vi "Write Scalar Data.vi"(8 "error in (no error)":errorcluster, 9 "Changed?":bool[](array[boolean]), 10 "Values":dbl[](array[numeric]), 11 "Cluster":T1 {"Data Type" format="%.0x"}) -> (0 "error out":errorcluster, 2 "Values":dbl[](array[numeric]), 3 "Cluster":T1 {"Data Type" format="%.0x"})   [LabVIEW 2017, in "FPGA Addon Engine.lvlib"]
uses:
  FPGA Addon Engine.lvlib
  Types/Register Settings.ctl
  Shared/Data Type.ctl
  Shared/Scalar Type.ctl
  <vilib>/rvi/errors/niLvFpgaAdjustHostInterfaceError.vi
  <vilib>/Utility/error.llb/Error Cluster From Error Code.vi
  <vilib>/rvi/interface/nirviReadWriteControl/nirviReadWriteControl.xnode
  <vilib>/rvi/interface/Simulation/niFpgaSimulationCallBeginRW.vi
  NiFpgaLv.dll
  Shared/FPGA Addon Shared.lvlib
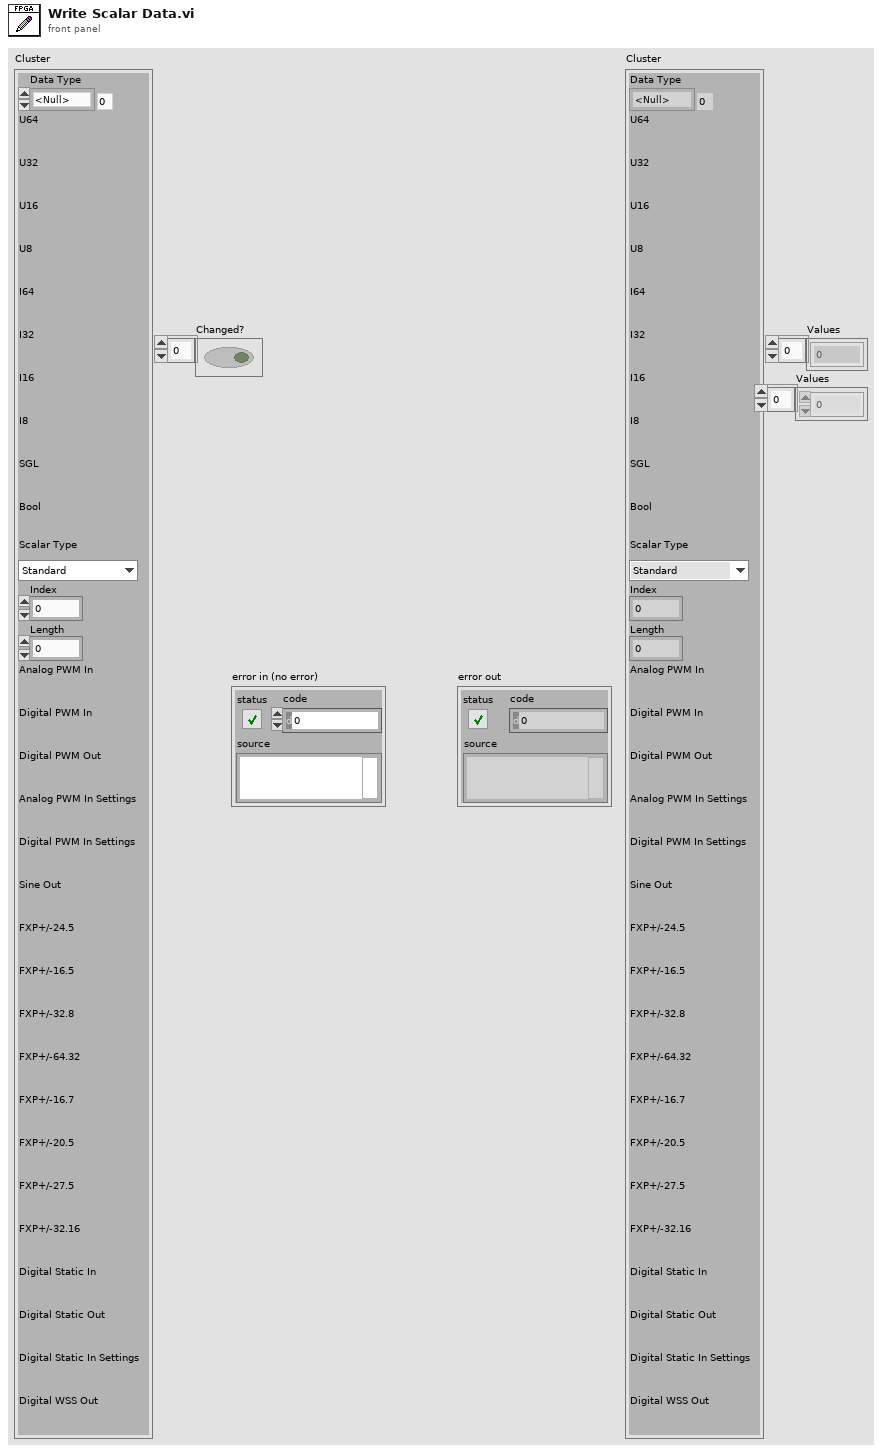
[diagram p1: front panel]
types:
  T1 = typedef "FPGA Addon Engine.lvlib/Register Settings.ctl" = cluster{"Data Type":T2, "U64":refnum<k20>, "U32":refnum<k20>, "U16":refnum<k20>, "U8":refnum<k20>, "I64":refnum<k20>, "I32":refnum<k20>, "I16":refnum<k20>, "I8":refnum<k20>, "SGL":refnum<k20>, "Bool":refnum<k20>, "Scalar Type":T3, "Index":i32, "Length":i32, "Analog PWM In":refnum<k20>, "Digital PWM In":refnum<k20>, "Digital PWM Out":refnum<k20>, "Analog PWM In Settings":refnum<k20>, "Digital PWM In Settings":refnum<k20>, "Sine Out":refnum<k20>, "FXP+/-24.5":refnum<k20>, "FXP+/-16.5":refnum<k20>, "FXP+/-32.8":refnum<k20>, "FXP+/-64.32":refnum<k20>, "FXP+/-16.7":refnum<k20>, "FXP+/-20.5":refnum<k20>, "FXP+/-27.5":refnum<k20>, "FXP+/-32.16":refnum<k20>, "Digital Static In":refnum<k20>, "Digital Static Out":refnum<k20>, "Digital Static In Settings":refnum<k20>, "Digital WSS Out":refnum<k20>}
  T2 = typedef "FPGA Addon Shared.lvlib/Data Type.ctl" = enum8{"<Null>", "I8", "I16", "I32", "I64", "U8", "U16", "U32", "U64", "SGL", "Boolean", "Analog PWM In Settings", "Analog PWM In", "Digital PWM In Settings", "Digital PWM In", "Digital PWM Out", "Sine Out", "FXP+/-24.5", "FXP+/-16.5", "FXP+/-32.8", "FXP+/-64.32", "FXP+/-16.7", "FXP+/-20.5", "FXP+/-27.5", "FXP+/-32.16", "Digital Static In", "Digital Static Out", "Digital Static In Settings", "Digital WSS Out"}
  T3 = typedef "FPGA Addon Shared.lvlib/Scalar Type.ctl" = enum16{"Standard", "Bitpacked"}
  T4 = cluster{"ACTIVE EDGE":bool, "TIMEOUT":u32, "THRESHOLD":fxp<+/-,32,8>}
  T5 = cluster{"ACTIVE EDGE":bool, "ACTIVE TICKS":u32, "INACTIVE TICKS":u32}
  T6 = cluster{"ACTIVE EDGE":bool, "ACTIVE TICKS":u32, "INACTIVE TICKS":u32, "DATA":u8, "SENSOR TYPE":u8}
  T7 = cluster{"AMP":fxp<+/-,32,8>, "OFFSET":fxp<+/-,32,8>, "PERIODS/TICKS":fxp<+,32,0>}
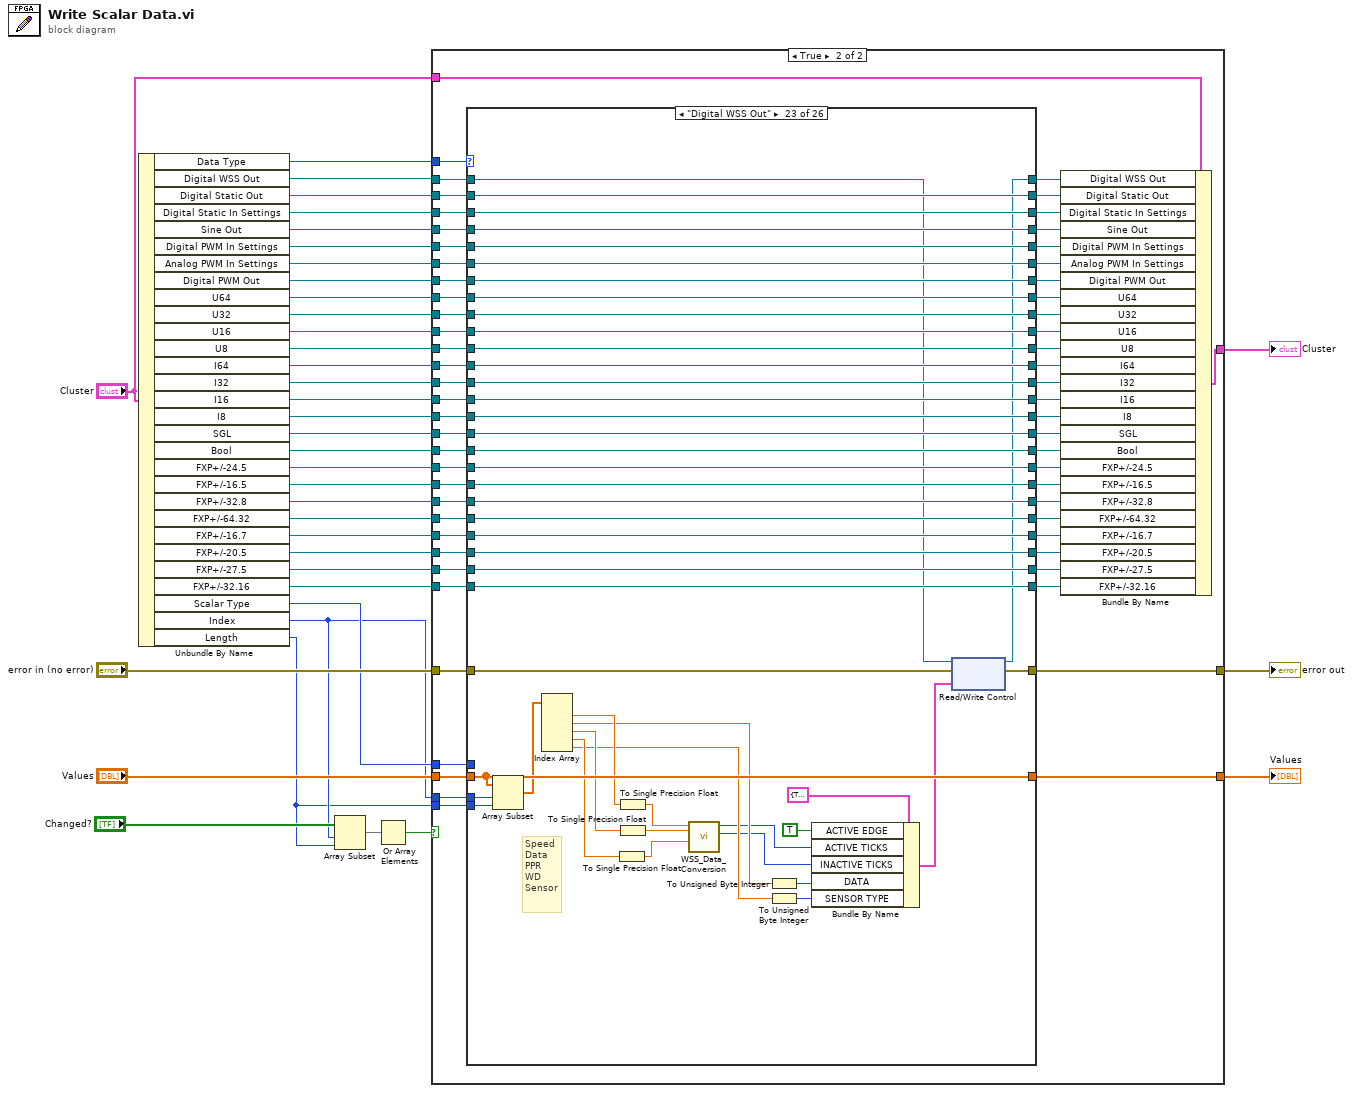
[diagram p0: block diagram]
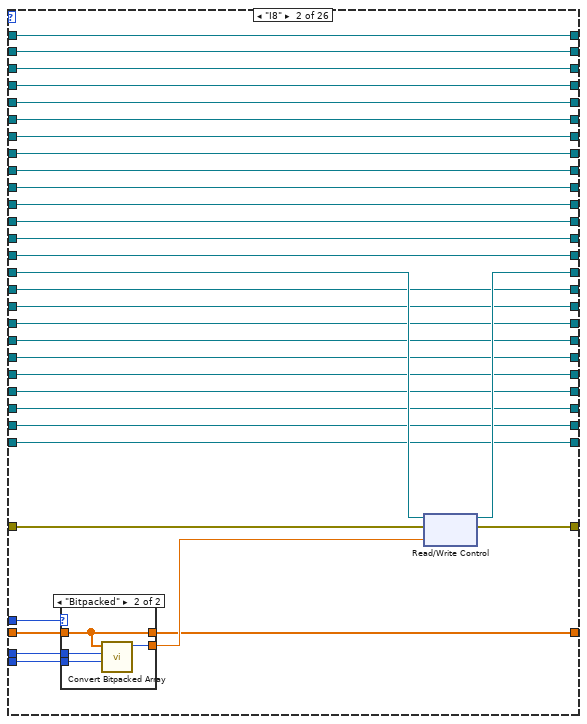
[diagram p4: hidden frame]
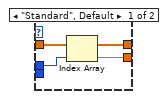
[diagram p5: hidden frame]
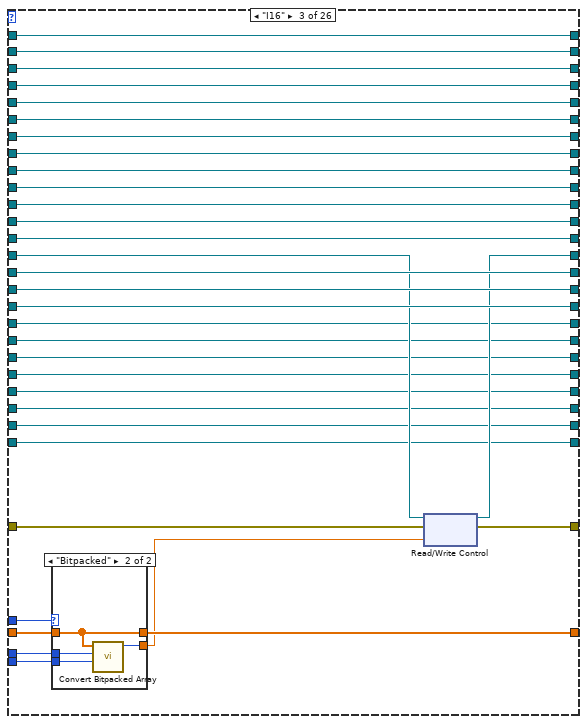
[diagram p6: hidden frame]
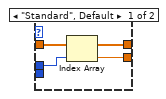
[diagram p7: hidden frame]
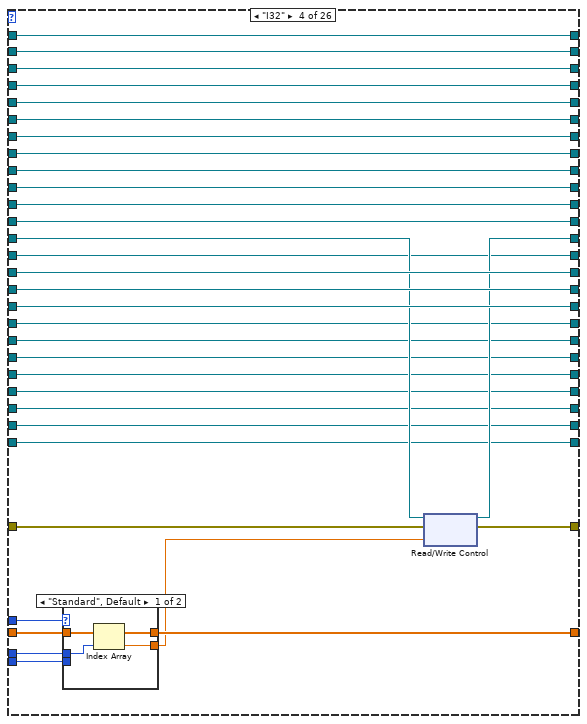
[diagram p8: hidden frame]
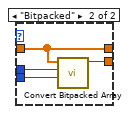
[diagram p9: hidden frame]
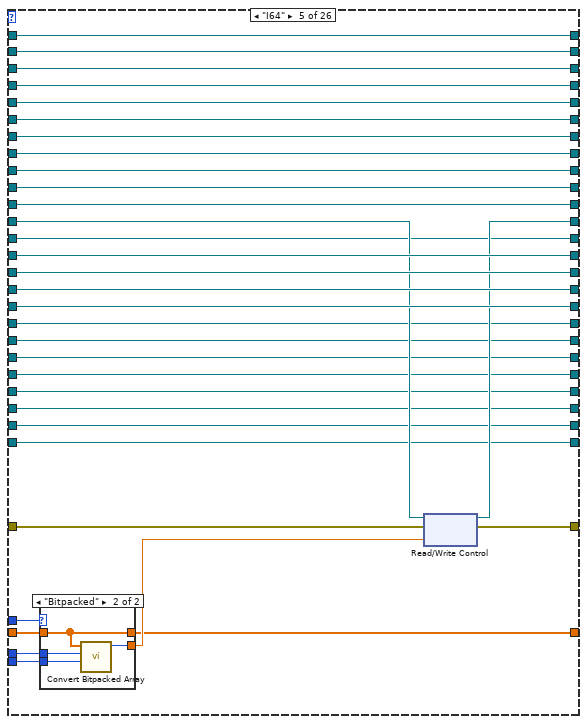
[diagram p10: hidden frame]
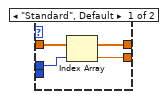
[diagram p11: hidden frame]
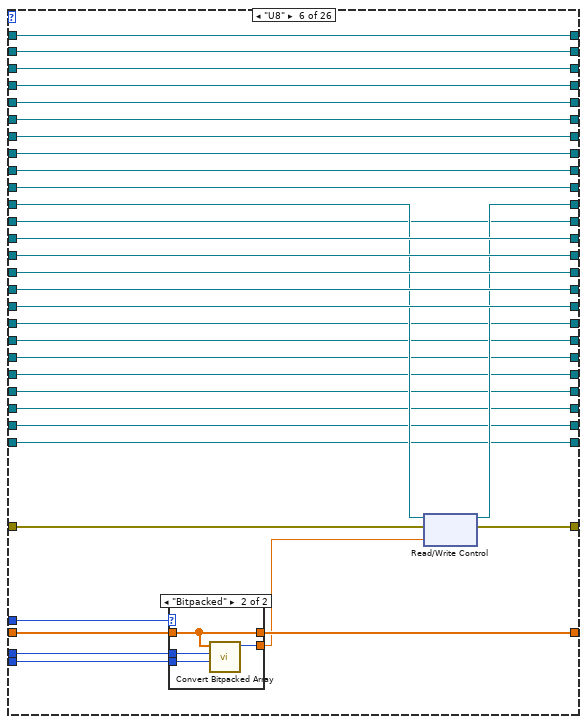
[diagram p12: hidden frame]
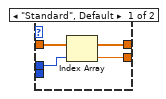
[diagram p13: hidden frame]
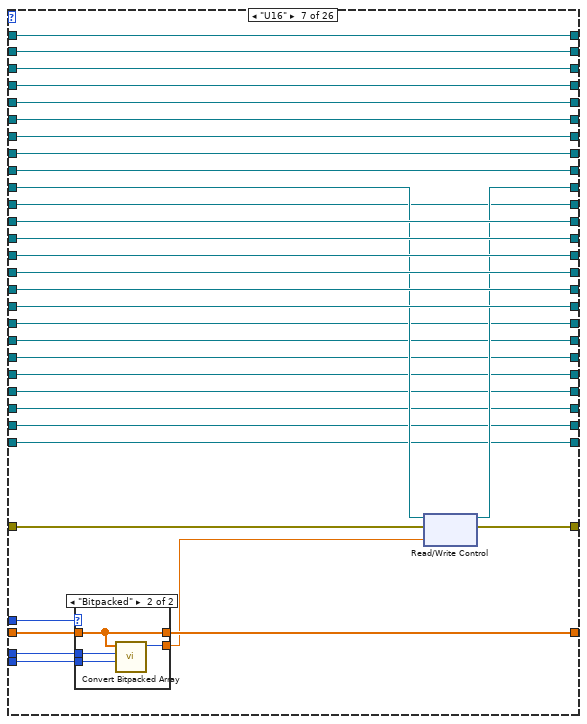
[diagram p14: hidden frame]
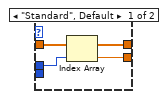
[diagram p15: hidden frame]
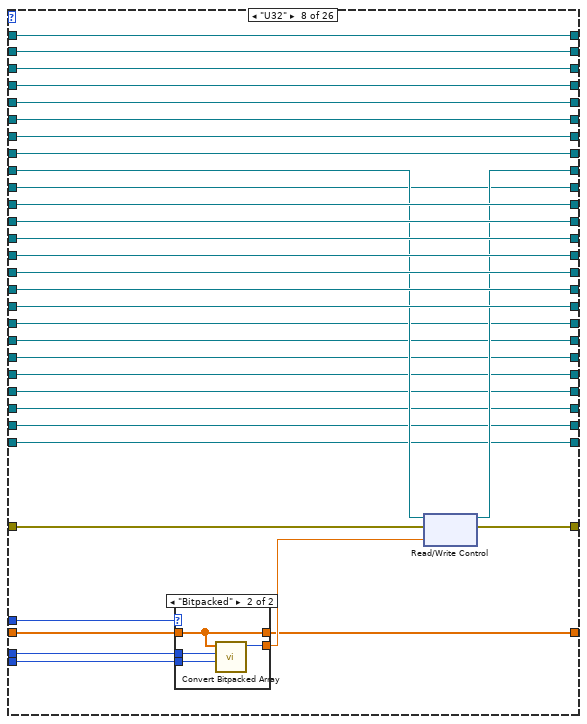
[diagram p16: hidden frame]
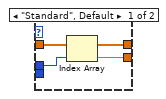
[diagram p17: hidden frame]
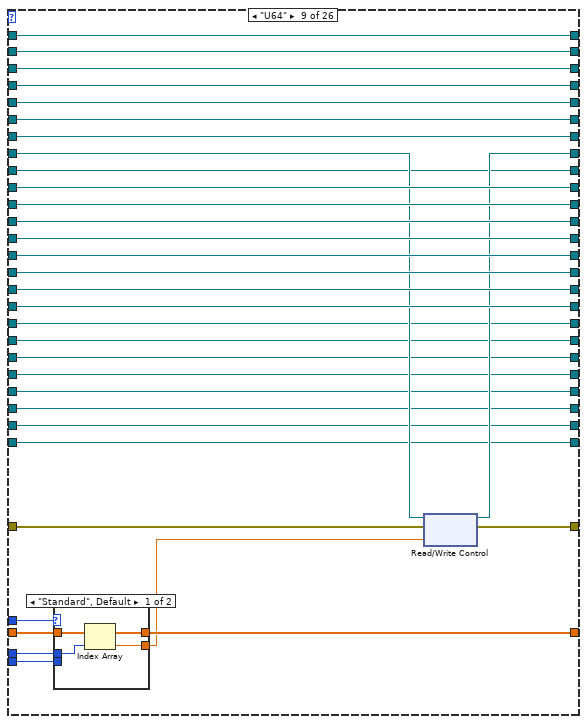
[diagram p18: hidden frame]
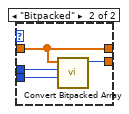
[diagram p19: hidden frame]
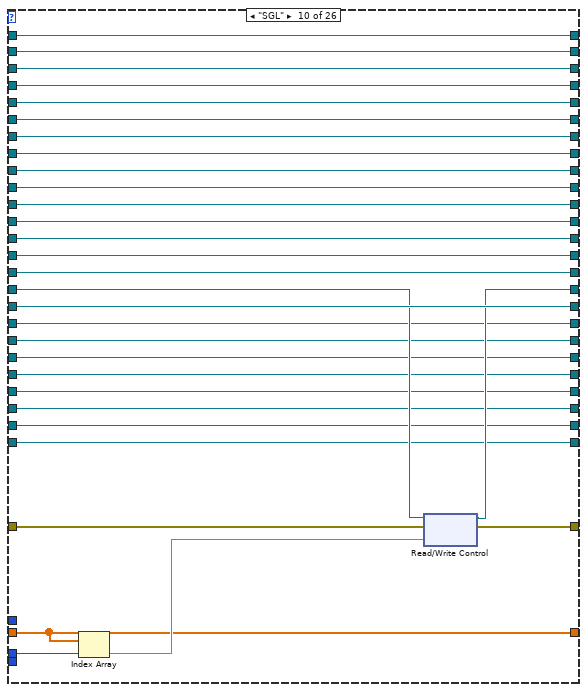
[diagram p20: hidden frame]
diagram:
  n1 = Unbundle By Name("Cluster") -> ("Data Type"=w1:T2, "Digital WSS Out"=w2:refnum<k20>, "Digital Static Out"=w4:refnum<k20>, "Digital Static In Settings"=w3:refnum<k20>, "Sine Out"=w13:refnum<k20>, "Digital PWM In Settings"=w19:refnum<k20>, "Analog PWM In Settings"=w20:refnum<k20>, "Digital PWM Out"=w21:refnum<k20>, "U64"=w26:refnum<k20>, "U32"=w27:refnum<k20>, "U16"=w28:refnum<k20>, "U8"=w29:refnum<k20>, "I64"=w30:refnum<k20>, "I32"=w31:refnum<k20>, "I16"=w32:refnum<k20>, "I8"=w38:refnum<k20>, "SGL"=w34:refnum<k20>, "Bool"=w33:refnum<k20>, "FXP+/-24.5"=w9:refnum<k20>, "FXP+/-16.5"=w10:refnum<k20>, "FXP+/-32.8"=w11:refnum<k20>, "FXP+/-64.32"=w12:refnum<k20>, "FXP+/-16.7"=w8:refnum<k20>, "FXP+/-20.5"=w7:refnum<k20>, "FXP+/-27.5"=w6:refnum<k20>, "FXP+/-32.16"=w5:refnum<k20>, "Scalar Type"=w22:T3, "Index"=w17:i32, "Length"=w16:i32)
  n2 = Array Subset(array="Changed?", index=w17, length=w16) -> (w15:bool[])
  n3 = Or Array Elements(Boolean array=w15) -> (logical OR=w14:bool)
  n4 = case shown="True" w14 {
    tunnel: w1 -> [_ w101]
    tunnel: w38 -> [_ w100]
    tunnel: "error in (no error)" -> [w40 w99]
    tunnel: [w40 w98] -> w36
    tunnel: "Cluster" -> [w41 w97]
    tunnel: w34 -> [_ w94]
    tunnel: w33 -> [_ w93]
    tunnel: w32 -> [_ w90]
    tunnel: w31 -> [_ w88]
    tunnel: w30 -> [_ w86]
    tunnel: w29 -> [_ w84]
    tunnel: w28 -> [_ w82]
    tunnel: w27 -> [_ w80]
    tunnel: w26 -> [_ w78]
    tunnel: [w41 w77] -> w25
    tunnel: [w39 w76] -> w24
    tunnel: "Values" -> [w39 w75]
    tunnel: w22 -> [_ w74]
    tunnel: w21 -> [_ w72]
    tunnel: w20 -> [_ w71]
    tunnel: w19 -> [_ w68]
    tunnel: w17 -> [_ w67]
    tunnel: w16 -> [_ w66]
    tunnel: w13 -> [_ w65]
    tunnel: w12 -> [_ w62]
    tunnel: w11 -> [_ w61]
    tunnel: w10 -> [_ w58]
    tunnel: w9 -> [_ w57]
    tunnel: w8 -> [_ w55]
    tunnel: w7 -> [_ w53]
    tunnel: w6 -> [_ w51]
    tunnel: w5 -> [_ w49]
    tunnel: w4 -> [_ w47]
    tunnel: w3 -> [_ w44]
    tunnel: w2 -> [_ w43]
    frame False {
    }
    frame True {
      n5 = case shown="\"Digital WSS Out\"" w101 {
        tunnel: w100 -> [w126 w162 w193 w235 w277 w319 w361 w403 w445 w484 w518 w549 w580 w611 w642 w673 w704 w735 w766 w798 w837 w899 w949 w988 w1025 w1064]
        tunnel: w99 -> [w118 w161 w203 w244 w285 w326 w367 w408 w449 w487 w520 w551 w582 w613 w644 w675 w706 w737 w768 w795 w834 w887 w937 w976 w997 w1052]
        tunnel: [w118 w160 w202 w243 w284 w325 w366 w407 w448 w486 w519 w550 w581 w612 w643 w674 w705 w736 w767 w794 w833 w886 w936 w975 w998 w1051] -> w98
        tunnel: [w126 w159 w193 w235 w277 w319 w361 w403 w445 w484 w518 w549 w580 w611 w642 w673 w704 w735 w766 w798 w837 w899 w949 w988 w1025 w1064] -> w96
        tunnel: [w127 w158 w201 w242 w283 w324 w365 w406 w447 w475 w508 w541 w572 w603 w634 w665 w696 w727 w758 w797 w836 w898 w948 w987 w1024 w1063] -> w95
        tunnel: w94 -> [w127 w158 w201 w242 w283 w324 w365 w406 w447 w477 w508 w541 w572 w603 w634 w665 w696 w727 w758 w797 w836 w898 w948 w987 w1024 w1063]
        tunnel: w93 -> [w128 w157 w200 w241 w282 w323 w364 w405 w446 w485 w510 w530 w562 w594 w626 w657 w689 w720 w751 w796 w835 w897 w947 w986 w1023 w1062]
        tunnel: [w128 w157 w200 w241 w282 w323 w364 w405 w446 w485 w509 w530 w562 w594 w626 w657 w689 w720 w751 w796 w835 w897 w947 w986 w1023 w1062] -> w92
        tunnel: [w125 w156 w191 w232 w276 w318 w360 w402 w444 w483 w517 w548 w579 w610 w641 w672 w703 w734 w765 w799 w838 w896 w946 w985 w1022 w1061] -> w91
        tunnel: w90 -> [w125 w156 w192 w232 w276 w318 w360 w402 w444 w483 w517 w548 w579 w610 w641 w672 w703 w734 w765 w799 w838 w896 w946 w985 w1022 w1061]
        tunnel: [w124 w155 w199 w233 w273 w317 w359 w401 w443 w482 w516 w547 w578 w609 w640 w671 w702 w733 w764 w800 w839 w895 w945 w984 w1021 w1060] -> w89
        tunnel: w88 -> [w124 w155 w199 w234 w273 w317 w359 w401 w443 w482 w516 w547 w578 w609 w640 w671 w702 w733 w764 w800 w839 w895 w945 w984 w1021 w1060]
        tunnel: [w123 w154 w198 w240 w274 w314 w358 w400 w442 w481 w515 w546 w577 w608 w639 w670 w701 w732 w763 w801 w840 w894 w944 w983 w1020 w1059] -> w87
        tunnel: w86 -> [w123 w154 w198 w240 w275 w314 w358 w400 w442 w481 w515 w546 w577 w608 w639 w670 w701 w732 w763 w801 w840 w894 w944 w983 w1020 w1059]
        tunnel: [w122 w153 w197 w239 w281 w315 w355 w399 w441 w480 w514 w545 w576 w607 w638 w669 w700 w731 w762 w802 w841 w893 w943 w982 w1019 w1058] -> w85
        tunnel: w84 -> [w122 w153 w197 w239 w281 w316 w355 w399 w441 w480 w514 w545 w576 w607 w638 w669 w700 w731 w762 w802 w841 w893 w943 w982 w1019 w1058]
        tunnel: [w121 w152 w196 w238 w280 w322 w356 w396 w440 w479 w513 w544 w575 w606 w637 w668 w699 w730 w761 w803 w842 w892 w942 w981 w1018 w1057] -> w83
        tunnel: w82 -> [w121 w152 w196 w238 w280 w322 w357 w396 w440 w479 w513 w544 w575 w606 w637 w668 w699 w730 w761 w803 w842 w892 w942 w981 w1018 w1057]
        tunnel: [w120 w151 w195 w237 w279 w321 w363 w397 w437 w478 w512 w543 w574 w605 w636 w667 w698 w729 w760 w804 w843 w891 w941 w980 w1017 w1056] -> w81
        tunnel: w80 -> [w120 w151 w195 w237 w279 w321 w363 w398 w437 w478 w512 w543 w574 w605 w636 w667 w698 w729 w760 w804 w843 w891 w941 w980 w1017 w1056]
        tunnel: [w119 w150 w194 w236 w278 w320 w362 w404 w438 w476 w511 w542 w573 w604 w635 w666 w697 w728 w759 w805 w844 w890 w940 w979 w1016 w1055] -> w79
        tunnel: w78 -> [w119 w150 w194 w236 w278 w320 w362 w404 w439 w476 w511 w542 w573 w604 w635 w666 w697 w728 w759 w805 w844 w890 w940 w979 w1016 w1055]
        tunnel: [w117 w144 w186 w227 w267 w309 w350 w390 w432 w472 w505 w540 w571 w602 w633 w664 w695 w726 w757 w789 w830 w880 w935 w974 w1013 w1050] -> w76
        tunnel: w75 -> [w117 w149 w190 w231 w272 w313 w354 w395 w436 w472 w505 w540 w571 w602 w633 w664 w695 w726 w757 w789 w830 w880 w935 w974 w1013 w1050]
        tunnel: w66 -> [_ w147 w188 w228 w269 w312 w352 w393 w433 _ _ _ _ _ _ _ _ _ _ w790 w831 w879 w934 w973 w1012 w1049]
        tunnel: w74 -> [_ w146 w187 w230 w271 w310 w351 w392 w435 _ _ _ _ _ _ _ _ _ _ _ _ _ _ _ _ _]
        tunnel: w67 -> [_ w148 w189 w229 w270 w311 w353 w394 w434 w474 w504 w539 w570 w601 w632 w663 w694 w725 w756 w791 w832 w878 w933 w972 w1011 w1048]
        tunnel: [w116 w141 w182 w223 w264 w305 w346 w387 w428 w469 w500 w536 w567 w598 w629 w660 w691 w722 w753 w807 w845 w884 w919 w968 w1010 w1046] -> w73
        tunnel: w72 -> [w116 w141 w182 w223 w264 w305 w346 w387 w428 w469 w500 w536 w567 w598 w629 w660 w691 w722 w753 w807 w845 w885 w919 w968 w1010 w1046]
        tunnel: w71 -> [w115 w142 w183 w224 w265 w306 w347 w388 w429 w470 w501 w537 w568 w599 w630 w661 w692 w723 w754 w793 w824 w889 w939 w978 w1015 w1054]
        tunnel: [w115 w142 w183 w224 w265 w306 w347 w388 w429 w470 w501 w537 w568 w599 w630 w661 w692 w723 w754 w792 w824 w889 w939 w978 w1015 w1054] -> w70
        tunnel: [w114 w143 w184 w225 w266 w307 w348 w389 w430 w471 w502 w538 w569 w600 w631 w662 w693 w724 w755 w806 w826 w888 w938 w977 w1014 w1053] -> w69
        tunnel: w68 -> [w114 w143 w184 w225 w266 w307 w348 w389 w430 w471 w502 w538 w569 w600 w631 w662 w693 w724 w755 w806 w825 w888 w938 w977 w1014 w1053]
        tunnel: w65 -> [w113 w140 w181 w222 w263 w304 w345 w386 w427 w468 w499 w535 w566 w597 w628 w659 w690 w721 w752 w782 w821 w859 w931 w970 w995 w1037]
        tunnel: [w113 w140 w181 w222 w263 w304 w345 w386 w427 w468 w499 w535 w566 w597 w628 w659 w690 w721 w752 w782 w821 w859 w931 w969 w995 w1037] -> w64
        tunnel: [w112 w139 w180 w221 w262 w303 w344 w385 w426 w467 w498 w534 w565 w596 w621 w653 w685 w716 w747 w781 w818 w856 w929 w960 w1009 w1045] -> w63
        tunnel: w62 -> [w112 w139 w180 w221 w262 w303 w344 w385 w426 w467 w498 w534 w565 w596 w623 w653 w685 w716 w747 w781 w818 w856 w929 w960 w1009 w1045]
        tunnel: w61 -> [w111 w138 w179 w220 w261 w302 w343 w384 w425 w466 w497 w533 w564 w590 w622 w654 w686 w717 w748 w780 w817 w855 w928 w959 w1008 w1044]
        tunnel: [w111 w138 w179 w220 w261 w302 w343 w384 w425 w466 w497 w533 w564 w591 w622 w654 w686 w717 w748 w780 w817 w855 w928 w959 w1008 w1044] -> w60
        tunnel: [w110 w137 w178 w219 w260 w301 w342 w383 w424 w465 w496 w532 w559 w592 w624 w655 w687 w718 w749 w779 w816 w854 w927 w958 w1007 w1043] -> w59
        tunnel: w58 -> [w110 w137 w178 w219 w260 w301 w342 w383 w424 w465 w496 w532 w560 w592 w624 w655 w687 w718 w749 w779 w816 w854 w927 w958 w1007 w1043]
        tunnel: w57 -> [w109 w136 w177 w218 w259 w300 w341 w382 w423 w464 w495 w529 w561 w593 w625 w656 w688 w719 w750 w778 w815 w853 w926 w957 w1006 w1042]
        tunnel: [w109 w136 w177 w218 w259 w300 w341 w382 w423 w464 w495 w528 w561 w593 w625 w656 w688 w719 w750 w778 w815 w853 w926 w957 w1006 w1042] -> w56
        tunnel: w55 -> [w108 w135 w176 w217 w258 w299 w340 w381 w422 w463 w494 w527 w558 w589 w620 w652 w683 w715 w746 w777 w814 w852 w925 w956 w1005 w1041]
        tunnel: [w108 w135 w176 w217 w258 w299 w340 w381 w422 w463 w494 w527 w558 w589 w620 w651 w683 w715 w746 w777 w814 w852 w925 w956 w1005 w1041] -> w54
        tunnel: w53 -> [w107 w134 w175 w216 w257 w298 w339 w380 w421 w462 w493 w526 w557 w588 w619 w650 w684 w712 w744 w774 w813 w851 w924 w955 w1004 w1040]
        tunnel: [w107 w134 w175 w216 w257 w298 w339 w380 w421 w462 w493 w526 w557 w588 w619 w650 w682 w712 w744 w774 w813 w851 w924 w955 w1004 w1040] -> w52
        tunnel: w51 -> [w106 w133 w174 w215 w256 w297 w338 w379 w420 w461 w492 w525 w556 w587 w618 w649 w680 w713 w741 w773 w812 w850 w923 w954 w1003 w1039]
        tunnel: [w106 w133 w174 w215 w256 w297 w338 w379 w420 w461 w492 w525 w556 w587 w618 w649 w680 w711 w741 w773 w812 w850 w923 w954 w1003 w1039] -> w50
        tunnel: w49 -> [w105 w132 w173 w214 w255 w296 w337 w378 w419 w460 w491 w524 w555 w586 w617 w648 w679 w710 w743 w772 w811 w849 w922 w953 w1002 w1038]
        tunnel: [w105 w132 w173 w214 w255 w296 w337 w378 w419 w460 w491 w524 w555 w586 w617 w648 w679 w710 w742 w772 w811 w849 w922 w953 w1002 w1038] -> w48
        tunnel: w47 -> [w104 w131 w172 w213 w254 w295 w336 w377 w418 w459 w490 w523 w554 w585 w616 w647 w678 w709 w740 w771 w810 w848 w921 w952 w990 w1035]
        tunnel: [w104 w131 w172 w213 w254 w295 w336 w377 w418 w459 w490 w523 w554 w585 w616 w647 w678 w709 w740 w771 w810 w848 w921 w952 w990 w1034] -> w46
        tunnel: [w103 w130 w171 w212 w253 w294 w335 w376 w417 w458 w489 w522 w553 w584 w615 w646 w677 w708 w739 w770 w809 w847 w920 w951 w991 w1036] -> w45
        tunnel: w44 -> [w103 w130 w171 w212 w253 w294 w335 w376 w417 w458 w489 w522 w553 w584 w615 w646 w677 w708 w739 w770 w809 w847 w920 w951 w994 w1036]
        tunnel: w43 -> [w102 w129 w170 w211 w252 w293 w334 w375 w416 w457 w488 w521 w552 w583 w614 w645 w676 w707 w738 w769 w808 w846 w917 w950 w989 w1026]
        tunnel: [w102 w129 w170 w211 w252 w293 w334 w375 w416 w457 w488 w521 w552 w583 w614 w645 w676 w707 w738 w769 w808 w846 w918 w950 w989 w1026] -> w42
        frame "<Null>", Default {
        }
        frame "I8" {
          n6 = case shown="\"Bitpacked\"" w146 {
            tunnel: w149 -> [w163 w166]
            tunnel: w148 -> [w165 w169]
            tunnel: [w164 w167] -> w145
            tunnel: w147 -> [_ w168]
            tunnel: [w163 w166] -> w144
            frame "Standard", Default {
              n7 = Index Array(array=w163, index=w165) -> (element=w164:dbl)
            }
            frame "Bitpacked" {
              n8 = call "Convert Bitpacked Array.vi"("Length"=w168, "Index"=w169, "Values"=w166) -> ("Numeric"=w167:u64)  [unwired: 8 in]
            }
          }
          n9 = xnode "Read/Write Control"("FPGA VI Reference In"=w162, "error in"=w161, "Value"=w145) -> ("FPGA VI Reference Out"=w159:refnum<k20>, "error out"=w160:errorcluster)
        }
        frame "I16" {
          n10 = case shown="\"Bitpacked\"" w187 {
            tunnel: w190 -> [w204 w207]
            tunnel: w189 -> [w206 w210]
            tunnel: [w205 w208] -> w185
            tunnel: w188 -> [_ w209]
            tunnel: [w204 w207] -> w186
            frame "Standard", Default {
              n11 = Index Array(array=w204, index=w206) -> (element=w205:dbl)
            }
            frame "Bitpacked" {
              n12 = call "Convert Bitpacked Array.vi"("Length"=w209, "Index"=w210, "Values"=w207) -> ("Numeric"=w208:u64)  [unwired: 8 in]
            }
          }
          n13 = xnode "Read/Write Control"("FPGA VI Reference In"=w192, "error in"=w203, "Value"=w185) -> ("FPGA VI Reference Out"=w191:refnum<k20>, "error out"=w202:errorcluster)
        }
        frame "I32" {
          n14 = case shown="\"Standard\", Default" w230 {
            tunnel: w231 -> [w245 w248]
            tunnel: w229 -> [w247 w251]
            tunnel: [w246 w249] -> w226
            tunnel: w228 -> [_ w250]
            tunnel: [w245 w248] -> w227
            frame "Standard", Default {
              n15 = Index Array(array=w245, index=w247) -> (element=w246:dbl)
            }
            frame "Bitpacked" {
              n16 = call "Convert Bitpacked Array.vi"("Length"=w250, "Index"=w251, "Values"=w248) -> ("Numeric"=w249:u64)  [unwired: 8 in]
            }
          }
          n17 = xnode "Read/Write Control"("FPGA VI Reference In"=w234, "error in"=w244, "Value"=w226) -> ("FPGA VI Reference Out"=w233:refnum<k20>, "error out"=w243:errorcluster)
        }
        frame "I64" {
          n18 = case shown="\"Bitpacked\"" w271 {
            tunnel: w272 -> [w286 w289]
            tunnel: w270 -> [w288 w292]
            tunnel: [w287 w290] -> w268
            tunnel: w269 -> [_ w291]
            tunnel: [w286 w289] -> w267
            frame "Standard", Default {
              n19 = Index Array(array=w286, index=w288) -> (element=w287:dbl)
            }
            frame "Bitpacked" {
              n20 = call "Convert Bitpacked Array.vi"("Length"=w291, "Index"=w292, "Values"=w289) -> ("Numeric"=w290:u64)  [unwired: 8 in]
            }
          }
          n21 = xnode "Read/Write Control"("FPGA VI Reference In"=w275, "error in"=w285, "Value"=w268) -> ("FPGA VI Reference Out"=w274:refnum<k20>, "error out"=w284:errorcluster)
        }
        frame "U8" {
          n22 = case shown="\"Bitpacked\"" w310 {
            tunnel: w313 -> [w327 w330]
            tunnel: w311 -> [w329 w333]
            tunnel: [w328 w331] -> w308
            tunnel: w312 -> [_ w332]
            tunnel: [w327 w330] -> w309
            frame "Standard", Default {
              n23 = Index Array(array=w327, index=w329) -> (element=w328:dbl)
            }
            frame "Bitpacked" {
              n24 = call "Convert Bitpacked Array.vi"("Length"=w332, "Index"=w333, "Values"=w330) -> ("Numeric"=w331:u64)  [unwired: 8 in]
            }
          }
          n25 = xnode "Read/Write Control"("FPGA VI Reference In"=w316, "error in"=w326, "Value"=w308) -> ("FPGA VI Reference Out"=w315:refnum<k20>, "error out"=w325:errorcluster)
        }
        frame "U16" {
          n26 = case shown="\"Bitpacked\"" w351 {
            tunnel: w354 -> [w368 w371]
            tunnel: w353 -> [w370 w374]
            tunnel: [w369 w372] -> w349
            tunnel: w352 -> [_ w373]
            tunnel: [w368 w371] -> w350
            frame "Standard", Default {
              n27 = Index Array(array=w368, index=w370) -> (element=w369:dbl)
            }
            frame "Bitpacked" {
              n28 = call "Convert Bitpacked Array.vi"("Length"=w373, "Index"=w374, "Values"=w371) -> ("Numeric"=w372:u64)  [unwired: 8 in]
            }
          }
          n29 = xnode "Read/Write Control"("FPGA VI Reference In"=w357, "error in"=w367, "Value"=w349) -> ("FPGA VI Reference Out"=w356:refnum<k20>, "error out"=w366:errorcluster)
        }
        frame "U32" {
          n30 = case shown="\"Bitpacked\"" w392 {
            tunnel: w395 -> [w409 w412]
            tunnel: w394 -> [w411 w415]
            tunnel: [w410 w413] -> w391
            tunnel: w393 -> [_ w414]
            tunnel: [w409 w412] -> w390
            frame "Standard", Default {
              n31 = Index Array(array=w409, index=w411) -> (element=w410:dbl)
            }
            frame "Bitpacked" {
              n32 = call "Convert Bitpacked Array.vi"("Length"=w414, "Index"=w415, "Values"=w412) -> ("Numeric"=w413:u64)  [unwired: 8 in]
            }
          }
          n33 = xnode "Read/Write Control"("FPGA VI Reference In"=w398, "error in"=w408, "Value"=w391) -> ("FPGA VI Reference Out"=w397:refnum<k20>, "error out"=w407:errorcluster)
        }
        frame "U64" {
          n34 = case shown="\"Standard\", Default" w435 {
            tunnel: w436 -> [w450 w453]
            tunnel: w434 -> [w452 w456]
            tunnel: [w451 w454] -> w431
            tunnel: w433 -> [_ w455]
            tunnel: [w450 w453] -> w432
            frame "Standard", Default {
              n35 = Index Array(array=w450, index=w452) -> (element=w451:dbl)
            }
            frame "Bitpacked" {
              n36 = call "Convert Bitpacked Array.vi"("Length"=w455, "Index"=w456, "Values"=w453) -> ("Numeric"=w454:u64)  [unwired: 8 in]
            }
          }
          n37 = xnode "Read/Write Control"("FPGA VI Reference In"=w439, "error in"=w449, "Value"=w431) -> ("FPGA VI Reference Out"=w438:refnum<k20>, "error out"=w448:errorcluster)
        }
        frame "SGL" {
          n38 = Index Array(array=w472, index=w474) -> (element=w473:dbl)
          n39 = xnode "Read/Write Control"("FPGA VI Reference In"=w477, "error in"=w487, "Value"=w473) -> ("FPGA VI Reference Out"=w475:refnum<k20>, "error out"=w486:errorcluster)
        }
        frame "Boolean" {
          n40 = Index Array(array=w505, index=w504) -> (element=w503:dbl)
          n41 = To Unsigned Byte Integer(number=w503) -> (unsigned 8bit integer=w506:u8)
          n42 = Greater Than 0?(x=w506) -> (x > 0?=w507:bool)
          n43 = xnode "Read/Write Control"("FPGA VI Reference In"=w510, "error in"=w520, "Value"=w507) -> ("FPGA VI Reference Out"=w509:refnum<k20>, "error out"=w519:errorcluster)
        }
        frame "FXP+/-24.5" {
          n44 = Index Array(array=w540, index=w539) -> (element=w531:dbl)
          n45 = xnode "Read/Write Control"("FPGA VI Reference In"=w529, "error in"=w551, "Value"=w531) -> ("FPGA VI Reference Out"=w528:refnum<k20>, "error out"=w550:errorcluster)
        }
        frame "FXP+/-16.5" {
          n46 = Index Array(array=w571, index=w570) -> (element=w563:dbl)
          n47 = xnode "Read/Write Control"("FPGA VI Reference In"=w560, "error in"=w582, "Value"=w563) -> ("FPGA VI Reference Out"=w559:refnum<k20>, "error out"=w581:errorcluster)
        }
        frame "FXP+/-32.8" {
          n48 = Index Array(array=w602, index=w601) -> (element=w595:dbl)
          n49 = xnode "Read/Write Control"("FPGA VI Reference In"=w590, "error in"=w613, "Value"=w595) -> ("FPGA VI Reference Out"=w591:refnum<k20>, "error out"=w612:errorcluster)
        }
        frame "FXP+/-64.32" {
          n50 = Index Array(array=w633, index=w632) -> (element=w627:dbl)
          n51 = xnode "Read/Write Control"("FPGA VI Reference In"=w623, "error in"=w644, "Value"=w627) -> ("FPGA VI Reference Out"=w621:refnum<k20>, "error out"=w643:errorcluster)
        }
        frame "FXP+/-16.7" {
          n52 = Index Array(array=w664, index=w663) -> (element=w658:dbl)
          n53 = xnode "Read/Write Control"("FPGA VI Reference In"=w652, "error in"=w675, "Value"=w658) -> ("FPGA VI Reference Out"=w651:refnum<k20>, "error out"=w674:errorcluster)
        }
        frame "FXP+/-20.5" {
          n54 = Index Array(array=w695, index=w694) -> (element=w681:dbl)
          n55 = xnode "Read/Write Control"("FPGA VI Reference In"=w684, "error in"=w706, "Value"=w681) -> ("FPGA VI Reference Out"=w682:refnum<k20>, "error out"=w705:errorcluster)
        }
        frame "FXP+/-27.5" {
          n56 = Index Array(array=w726, index=w725) -> (element=w714:dbl)
          n57 = xnode "Read/Write Control"("FPGA VI Reference In"=w713, "error in"=w737, "Value"=w714) -> ("FPGA VI Reference Out"=w711:refnum<k20>, "error out"=w736:errorcluster)
        }
        frame "FXP+/-32.16" {
          n58 = Index Array(array=w757, index=w756) -> (element=w745:dbl)
          n59 = xnode "Read/Write Control"("FPGA VI Reference In"=w743, "error in"=w768, "Value"=w745) -> ("FPGA VI Reference Out"=w742:refnum<k20>, "error out"=w767:errorcluster)
        }
        frame "Analog PWM In Settings" {
          n60 = Array Subset(array=w789, index=w791, length=w790) -> (w788:dbl[])
          n61 = Index Array(array=w788) -> (element #1=w786:dbl, element #2=w784:dbl, element #3=w783:dbl)  [unwired: 4 in, 1 out]
          n62 = Greater?(x=w786, y=0.5) -> (0:w785:bool)
          n63 = Bundle By Name(cluster=T4 {"ACTIVE EDGE"=FALSE, "TIMEOUT"=0, "THRESHOLD"=0.0} ("Value"), "ACTIVE EDGE"=w785, "TIMEOUT"=w784, "THRESHOLD"=w783) -> (w775:T4)
          n64 = xnode "Read/Write Control"("FPGA VI Reference In"=w793, "error in"=w795, "Value"=w775) -> ("FPGA VI Reference Out"=w792:refnum<k20>, "error out"=w794:errorcluster)
        }
        frame "Digital PWM In Settings" {
          n65 = Array Subset(array=w830, index=w832, length=w831) -> (w829:dbl[])
          n66 = Index Array(array=w829) -> (element #1=w823:dbl, element #2=w822:dbl)  [unwired: 2 in]
          n67 = Greater?(x=w823, y=0.5) -> (0:w828:bool)
          n68 = Bundle By Name(cluster=cluster{"ACTIVE EDGE":bool, "TIMEOUT":u32} {"ACTIVE EDGE"=FALSE, "TIMEOUT"=0} ("Value"), "ACTIVE EDGE"=w828, "TIMEOUT"=w822) -> (w819:cluster{"ACTIVE EDGE":bool, "TIMEOUT":u32})
          n69 = xnode "Read/Write Control"("FPGA VI Reference In"=w825, "error in"=w834, "Value"=w819) -> ("FPGA VI Reference Out"=w826:refnum<k20>, "error out"=w833:errorcluster)
        }
        frame "Digital PWM Out" {
          n70 = Array Subset(array=w880, index=w878, length=w879) -> (w877:dbl[])
          n71 = Index Array(array=w877) -> (element #1=w872:dbl, element #2=w870:dbl, element #3=w871:dbl)  [unwired: 3 in]
          n72 = To Single Precision Float(number=w870) -> (single precision float=w864:sgl)
          n73 = To Single Precision Float(number=w871) -> (single precision float=w863:sgl)
          n74 = In Range and Coerce(upper limit=sgl 100.0, x=w863, lower limit=sgl 0.0) -> (coerced(x)=w862:sgl)  [unwired: 1 out]
          n75 = Equal To 0?(x=w864) -> (x = 0?=w869:bool)
          n76 = Divide(x=sgl 40000000.0 ("y"), y=w864) -> (x/y=w867:sgl)
          n77 = Multiply(x=w862, y=sgl 0.01 ("x")) -> (x*y=w865:sgl)
          n78 = case shown="True" w869 {
            tunnel: [w901 w902] -> w868
            tunnel: w867 -> [w901 _]
            tunnel: [w900 w902] -> w866
            tunnel: w865 -> [w900 _]
            frame False {
            }
            frame True {
              w902 = sgl 0.0
            }
          }
          n79 = Greater?(x=w872, y=0.5) -> (0:w875:bool)
          n80 = To Unsigned Long Integer(number=w868) -> (unsigned 32bit integer=w882:u32)
          n81 = Multiply(x=w868, y=w866) -> (x*y=w874:u32)
          n82 = Subtract(x=w882, y=w874) -> (x-y=w873:u32)
          n83 = Bundle By Name(cluster=T5 {"ACTIVE EDGE"=FALSE, "ACTIVE TICKS"=0, "INACTIVE TICKS"=0} ("Value"), "ACTIVE EDGE"=w875, "ACTIVE TICKS"=w874, "INACTIVE TICKS"=w873) -> (w857:T5)
          n84 = xnode "Read/Write Control"("FPGA VI Reference In"=w885, "error in"=w887, "Value"=w857) -> ("FPGA VI Reference Out"=w884:refnum<k20>, "error out"=w886:errorcluster)
        }
        frame "Digital WSS Out" {
          # "Speed\nData\nPPR\nWD\nSensor"
          n85 = Array Subset(array=w935, index=w933, length=w934) -> (w932:dbl[])
          n86 = Index Array(array=w932) -> (element #1=w915:dbl, element #2=w914:dbl, element #3=w913:dbl, element #4=w912:dbl, element #5=w911:dbl)  [unwired: 5 in]
          n87 = To Single Precision Float(number=w912) -> (single precision float=w906:sgl)
          n88 = To Single Precision Float(number=w915) -> (single precision float=w908:sgl)
          n89 = To Single Precision Float(number=w913) -> (single precision float=w907:sgl)
          n90 = call "WSS_Data_Conversion.vi"("WD"=w906, "PPR"=w907, "Speed"=w908) -> ("Inactive"=w904:u32, "Active"=w905:u32)  [unwired: 7 in]
          n91 = To Unsigned Byte Integer(number=w914) -> (unsigned 8bit integer=w909:u8)
          n92 = To Unsigned Byte Integer(number=w911) -> (unsigned 8bit integer=w910:u8)
          n93 = Bundle By Name(cluster=T6 {"ACTIVE EDGE"=TRUE, "ACTIVE TICKS"=0, "INACTIVE TICKS"=0, "DATA"=0, "SENSOR TYPE"=0} ("Settings"), "ACTIVE EDGE"=TRUE, "ACTIVE TICKS"=w905, "INACTIVE TICKS"=w904, "DATA"=w909, "SENSOR TYPE"=w910) -> (w930:T6)
          n94 = xnode "Read/Write Control"("FPGA VI Reference In"=w917, "error in"=w937, "Value"=w930) -> ("FPGA VI Reference Out"=w918:refnum<k20>, "error out"=w936:errorcluster)
        }
        frame "Sine Out" {
          n95 = Array Subset(array=w974, index=w972, length=w973) -> (w971:dbl[])
          n96 = Index Array(array=w971) -> (element #1=w964:dbl, element #2=w965:dbl, element #3=w966:dbl)  [unwired: 3 in]
          n97 = Divide(x=w966, y=sgl 40000000.0) -> (x/y=w963:dbl)
          n98 = Bundle By Name(cluster=T7 {"AMP"=0.0, "OFFSET"=0.0, "PERIODS/TICKS"=0.0} ("Value"), "AMP"=w964, "OFFSET"=w965, "PERIODS/TICKS"=w963) -> (w961:T7)
          n99 = xnode "Read/Write Control"("FPGA VI Reference In"=w970, "error in"=w976, "Value"=w961) -> ("FPGA VI Reference Out"=w969:refnum<k20>, "error out"=w975:errorcluster)
        }
        frame "Digital Static In Settings" {
          n100 = Array Subset(array=w1013, index=w1011, length=w1012) -> (w996:dbl[])
          n101 = Index Array(array=w996) -> (element=w1001:dbl)  [unwired: 1 in]
          n102 = Greater?(x=w1001, y=0.5) -> (0:w999:bool)
          n103 = Bundle By Name(cluster=cluster{"ACTIVE EDGE":bool} {"ACTIVE EDGE"=FALSE} ("Value"), "ACTIVE EDGE"=w999) -> (w992:cluster{"ACTIVE EDGE":bool})
          n104 = xnode "Read/Write Control"("FPGA VI Reference In"=w994, "error in"=w997, "Value"=w992) -> ("FPGA VI Reference Out"=w991:refnum<k20>, "error out"=w998:errorcluster)
        }
        frame "Digital Static Out" {
          w1031 = 0.5 ("y")
          n105 = Array Subset(array=w1050, index=w1048, length=w1049) -> (w1047:dbl[])
          n106 = Index Array(array=w1047) -> (element #1=w1032:dbl, element #2=w1030:dbl)  [unwired: 2 in]
          n107 = Greater?(x=w1032, y=w1031) -> (0:w1028:bool)
          n108 = Greater?(x=w1030, y=w1031) -> (0:w1029:bool)
          n109 = Bundle By Name(cluster=cluster{"ACTIVE EDGE":bool, "OUTPUT":bool} {"ACTIVE EDGE"=FALSE, "OUTPUT"=FALSE} ("Value"), "ACTIVE EDGE"=w1028, "OUTPUT"=w1029) -> (w1027:cluster{"ACTIVE EDGE":bool, "OUTPUT":bool})
          n110 = xnode "Read/Write Control"("FPGA VI Reference In"=w1035, "error in"=w1052, "Value"=w1027) -> ("FPGA VI Reference Out"=w1034:refnum<k20>, "error out"=w1051:errorcluster)
        }
      }
      n111 = Bundle By Name(cluster=w97, "Digital WSS Out"=w42, "Digital Static Out"=w46, "Digital Static In Settings"=w45, "Sine Out"=w64, "Digital PWM In Settings"=w69, "Analog PWM In Settings"=w70, "Digital PWM Out"=w73, "U64"=w79, "U32"=w81, "U16"=w83, "U8"=w85, "I64"=w87, "I32"=w89, "I16"=w91, "I8"=w96, "SGL"=w95, "Bool"=w92, "FXP+/-24.5"=w56, "FXP+/-16.5"=w59, "FXP+/-32.8"=w60, "FXP+/-64.32"=w63, "FXP+/-16.7"=w54, "FXP+/-20.5"=w52, "FXP+/-27.5"=w50, "FXP+/-32.16"=w48) -> (w77:T1)
    }
  }
  "error out" <- w36
  "Cluster" <- w25
  "Values" <- w24
